vi "RFSA Fetch.vi"(5 "RX Port":string, 6 "instrument handle":refnum<k15>, 7 "reference level (dBm)":dbl format="%.2f", 8 "error in (no error)":errorcluster, 9 "Frequency":dbl, 10 "Pin":string, 11 "Semiconductor Module Context":T1) -> (0 "error out":errorcluster, 3 "power spectrum":cluster{"f0":dbl, "df":dbl, "data":dbl[]})   [LabVIEW 2014]
uses:
  <vilib>/NI_TestStand_SemiconductorModule/NI_TestStand_Semiconductor_Module.lvlibp/PinMap/General/SemiconductorModuleContext.ctl
  <vilib>/NI_TestStand_SemiconductorModule/NI_TestStand_Semiconductor_Module.lvlibp/PinMap/RF/RFmx/PinToNIRFmxSession.vi
  <instrlib>/niRFSA/niRFSA.llb/niRFSA Configure Spectrum Frequency Center Span.vi
  <instrlib>/niRFPM/niRFPM.llb/NI-RFPM Set RX Path By Parameters.vi
  <instrlib>/niRFPM/niRFPM.llb/NI-RFPM Fetch Receiver Offset By Parameters.vi
  <vilib>/NI_TestStand_SemiconductorModule/NI_TestStand_Semiconductor_Module.lvlibp
  <vilib>/NI_TestStand_SemiconductorModule/NI_TestStand_Semiconductor_Module.lvlibp/PinMap/RF/RFSA/PinToNIRFSASession.vi
panel:
  out "Waveform Graph":cluster{"f0":dbl, "df":dbl, "data":dbl[]}(graph)
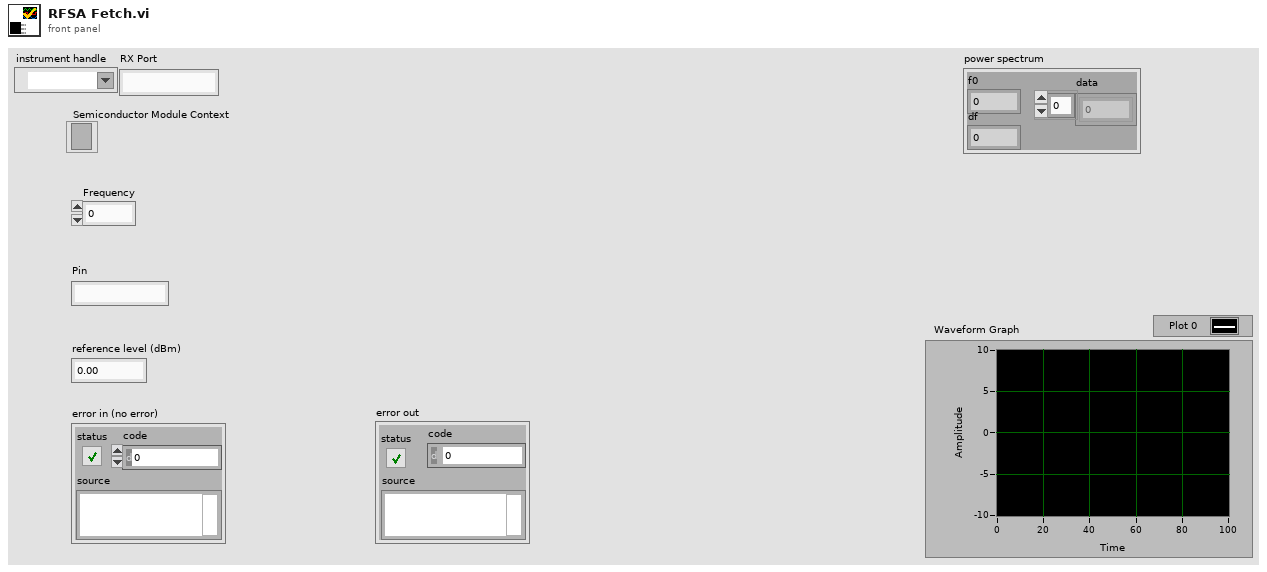
[diagram p1: front panel]
types:
  T1 = typedef "NI_TestStand_Semiconductor_Module.lvlibp/SemiconductorModuleContext.ctl" = refnum<k7>
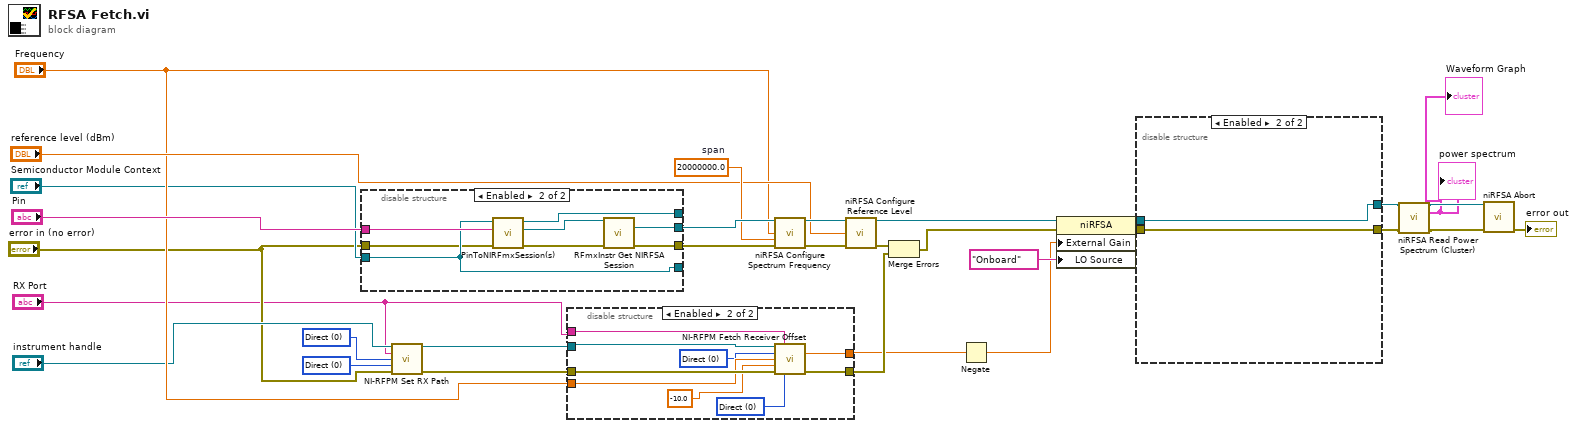
[diagram p0: block diagram]
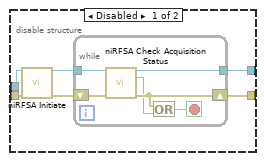
[diagram p2: hidden frame]
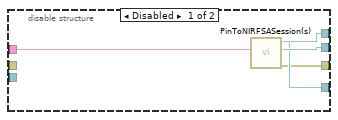
[diagram p3: hidden frame]
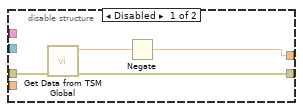
[diagram p4: hidden frame]
diagram:
  w20 = 0 items=["Direct", "Coupled", "LNA"] ("Receiver Coupling Path")
  w21 = 0 items=["Direct", "Gain", "Loop"] ("RX Path")
  w23 = 20000000.0  # span
  n1 = disable-structure shown="Enabled" {
    disable-tunnel: [w36 w41] -> w27
    disable-tunnel: [w35 w38] -> _
    disable-tunnel: [w34 w39] -> w26
    disable-tunnel: "Pin" -> [w33 w44]
    disable-tunnel: [w32 w43] -> _
    disable-tunnel: "Semiconductor Module Context" -> [_ w38]
    disable-tunnel: "error in (no error)" -> [_ w37]
    frame Disabled {
      n2 = call-poly <vilib>:"PinToNIRFSASession(s).vi"("Pin"=w33, "Semiconductor Module Context"=w35) -> ("error out"=w34:errorcluster, "Instrument Session"=w36:refnum<k15>, "Semiconductor Module Context Out"=w32:T1)  [unwired: 6 in, 1 out]
    }
    frame Enabled {
      n3 = call-poly <vilib>:"PinToNIRFmxSession(s).vi"("error in (no error)"=w37, "Pin"=w44, "Semiconductor Module Context"=w38) -> ("error out"=w40:errorcluster, "Instrument Session"=w42:refnum<k21>, "Semiconductor Module Context Out"=w43:T1)  [unwired: 5 in, 1 out]
      n4 = call <vilib>:"RFmxInstr Get NIRFSA Session.vi"("Instrument Handle In"=w42, "error in (no error)"=w40) -> ("NI RFSA Session"=w41:refnum<k15>, "error out"=w39:errorcluster)  [unwired: 11 in, 1 out]
    }
  }
  n5 = call-poly <instrlib>:"NI-RFPM Set RX Path.vi"("instrument handle"="instrument handle", "RX port"="RX Port", "RX Path"=w21, "Receiver Coupling Path"=w20, "error in (no error)"="error in (no error)") -> ("instrument handle out"=w19:refnum<k15>, "error out"=w12:errorcluster)  [unwired: 9 in]
  n6 = disable-structure shown="Enabled" {
    disable-tunnel: w12 -> [w48 w57]
    disable-tunnel: [w47 w56] -> w10
    disable-tunnel: [w45 w54] -> w7
    disable-tunnel: w19 -> [_ w55]
    disable-tunnel: "Frequency" -> [_ w53]
    disable-tunnel: "RX Port" -> [_ w51]
    frame Disabled {
      n7 = call "Get Data from TSM Global.vi"("error in (no error)"=w48) -> ("error out"=w47:errorcluster, "Look Up Value"=w46:dbl)  [unwired: 9 in]
      n8 = Negate(x=w46) -> (-x=w45:dbl)
    }
    frame Enabled {
      w50 = u32 0 items=["Unspecified"=3, "LNA"=2, "Direct"=0, "Coupled"=1] ("Receiver Coupling Path")
      w52 = u32 0 items=["Unspecified"=3, "Loop"=2, "Gain"=1, "Direct"=0] ("Receiver Path")
      n9 = call-poly <instrlib>:"NI-RFPM Fetch Receiver Offset.vi"("instrument handle"=w55, "Port"=w51, "Receiver Path"=w52, "frequency"=w53, "Reference Level"=-10.0, "error in"=w57, "Receiver Coupling Path"=w50) -> ("Receiver Offset"=w54:dbl, "error out"=w56:errorcluster)  [unwired: 4 in, 3 out]
    }
  }
  n10 = call-poly <instrlib>:"niRFSA Configure Spectrum Frequency.vi"("instrument handle"=w27, "frequency"="Frequency", "span"=w23, "error in"=w26) -> ("instrument handle out"=w25:refnum<k15>, "error out"=w24:errorcluster)  [unwired: 10 in]
  n11 = call <instrlib>:"niRFSA Configure Reference Level.vi"("instrument handle"=w25, "reference level (dBm)"="reference level (dBm)", "error in"=w24) -> ("instrument handle out"=w29:refnum<k15>, "error out"=w9:errorcluster)  [unwired: 11 in]
  n12 = Merge Errors(w9, w10) -> (w8:errorcluster)
  n13 = Negate(x=w7) -> (-x=w6:dbl)
  n14 = property class="niRFSA"(reference=w29, error in=w8, "External Gain"=w6, "LO Source"="Onboard" ("Signal Path:LO Source")) -> (reference out=w31:refnum<k15>, error out=w30:errorcluster)
  n15 = disable-structure shown="Enabled" {
    disable-tunnel: w31 -> [w61 w71]
    disable-tunnel: w30 -> [w60 w70]
    disable-tunnel: [w59 w71] -> w5
    disable-tunnel: [w58 w70] -> w4
    frame Disabled {
      n16 = call <instrlib>:"niRFSA Initiate.vi"("instrument handle"=w61, "error in"=w60) -> ("instrument handle out"=w63:refnum<k15>, "error out"=w62:errorcluster)  [unwired: 12 in]
      n17 = while {
        tunnel: w63 -> [w69]
        tunnel: [w67] -> w59
        shift-right: [w66] -> w58
        shift-left: w62 -> [w68]
        stop <- w64 stop-if-true
        n18 = call <instrlib>:"niRFSA Check Acquisition Status.vi"("instrument handle"=w69, "error in"=w68) -> ("instrument handle out"=w67:refnum<k15>, "done?"=w65:bool, "error out"=w66:errorcluster)  [unwired: 11 in]
        n19 = Or(x=w66, y=w65) -> (x .or. y?=w64:bool)
      }
    }
    frame Enabled {
    }
  }
  n20 = call <instrlib>:"niRFSA Read Power Spectrum (Cluster).vi"("instrument handle"=w5, "error in"=w4) -> ("instrument handle out"=w3:refnum<k15>, "power spectrum"=→"power spectrum" →"Waveform Graph":cluster{"f0":dbl, "df":dbl, "data":dbl[]}, "error out"=w2:errorcluster)  [unwired: 11 in]
  n21 = call <instrlib>:"niRFSA Abort.vi"("instrument handle"=w3, "error in"=w2) -> ("error out"=→"error out":errorcluster)  [unwired: 12 in, 1 out]
